vi "Destroy to Session.vi"(8 "Error In":errorcluster, 11 "Channel":refnum<class "Channel.lvclass">) -> (0 "Error Out":errorcluster, 3 "Session":refnum<class "Session.lvclass">)   [LabVIEW 2018, in "Toolkit.lvlib" / "Channel.lvclass"]
uses:
  Channel.lvclass
  Session/Session.lvclass
  Channel.lvclass/Channel.ctl
  Session/Session.lvclass/Session.ctl
  SSH/SSH.lvclass/SSH.ctl
  Toolkit.lvlib
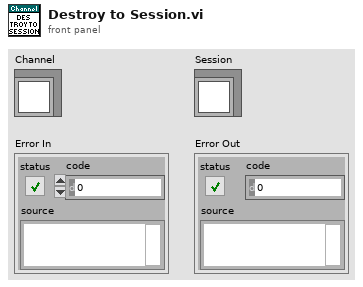
[diagram p1: front panel]
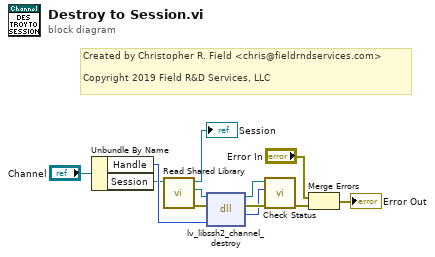
[diagram p0: block diagram]
diagram:
  # "Created by Christopher R. Field <chris@fieldrndservices.com>\n\nCopyright 2019 Field R&D Services, LLC"
  n1 = Unbundle By Name("Channel") -> ("Handle"=w10:u64, "Session"=w4:refnum<class "Session.lvclass">)
  n2 = call "Read Shared Library.vi"("Session In"=w4) -> ("Erorr Out"=w2:errorcluster, "libssh2lv Shared Library"=w3:path, "Session Out"=→"Session":refnum<class "Session.lvclass">)  [unwired: 8 in]
  n3 = dll-call lib="lv-libssh2.*" fn="lv_libssh2_channel_destroy"(path in=w3, error in=w2, "handle"=w10) -> (path out=w8:path, error out=w9:errorcluster, "status"=w7:i32)  [unwired: 2 in]
  n4 = call "Check Status.vi"("Error In"=w9, "Status"=w7, "lv-libssh2 Shared Library In"=w8) -> ("Error Out"=w6:errorcluster)  [unwired: 7 in, 1 out]
  n5 = Merge Errors("Error In", w6) -> (→"Error Out":errorcluster)
